vi "01b-add_two_numbers.vi"() -> ()   [LabVIEW 2018, in "LV-0mq-Julia_roundtrip-lib.lvlib"]
uses:
  LV-0mq-Julia_roundtrip-lib.lvlib
  Server or client state.ctl
  detailed error info.ctl
  StackFrame.ctl
  Commands.ctl
  d2cb43a9-9305-42fb-ad58-bce983510195.vi
  d2cb43a9-9305-42fb-ad58-bce983510195.vi/e28c4e1c-617d-4a26-8291-f58a5accd33d.vi
  d2cb43a9-9305-42fb-ad58-bce983510195.vi/697b26af-9cff-4296-98ec-fa9d12ca8fdc.vi
  d2cb43a9-9305-42fb-ad58-bce983510195.vi/17159f77-75f5-4b7b-8d47-844af2eb1bcd.vi
  jl-scripts path.vi
  check ID validity.vi
  bindata_descr to JSON.vi
  check cluster field names.vi
  concat JSON.vi
panel:
  in  "y":dbl=2.0
  in  "x":dbl=2.0
  in  "next":bool
  out "x+y":dbl=nan
  out "detailed error info":T1
  out "current error":errorcluster
  out "final error":errorcluster
  out "short err code":u8
  in  "stop":bool
  out "ZMQ timeout":bool
  out "Julia script file path":path
  out "temporary script path":path
  out "Jl Server state":T3
  # "This VI is slightly different from the previous example (see the wiring diagramm), but uses the same julia script."
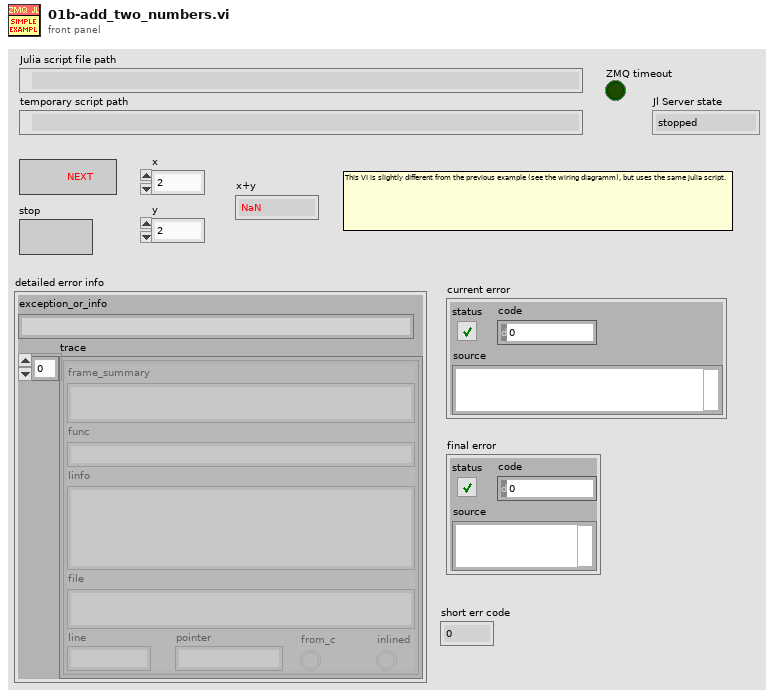
[diagram p1: front panel]
types:
  T1 = typedef "LV-0mq-Julia_roundtrip-lib.lvlib/detailed error info.ctl" = cluster{"exception_or_info":string, "trace":T2[]}
  T2 = typedef "LV-0mq-Julia_roundtrip-lib.lvlib/StackFrame.ctl" = cluster{"frame_summary":string, "func":string, "linfo":string, "file":string, "line":i32, "pointer":u64, "from_c":bool, "inlined":bool}
  T3 = typedef "LV-0mq-Julia_roundtrip-lib.lvlib/Server or client state.ctl" = enum16{"stopped", "running", "unknown"}
  T4 = typedef "LV-0mq-Julia_roundtrip-lib.lvlib/Commands.ctl" = enum16{"Start Jl-server & Init LV-client", "Send request & Get response ", "Stop Jl-server & Cleanup LV-client", "Cleanup LV-client", "Start Jl-server", "Stop Jl-server", "Init LV-Client", "Cleanup LV-Client", "(not allowed)", "Set LV Client state", "Set Jl Server state", "set ZMQ timeout", "read ZMQ timeout", "read-out state"}
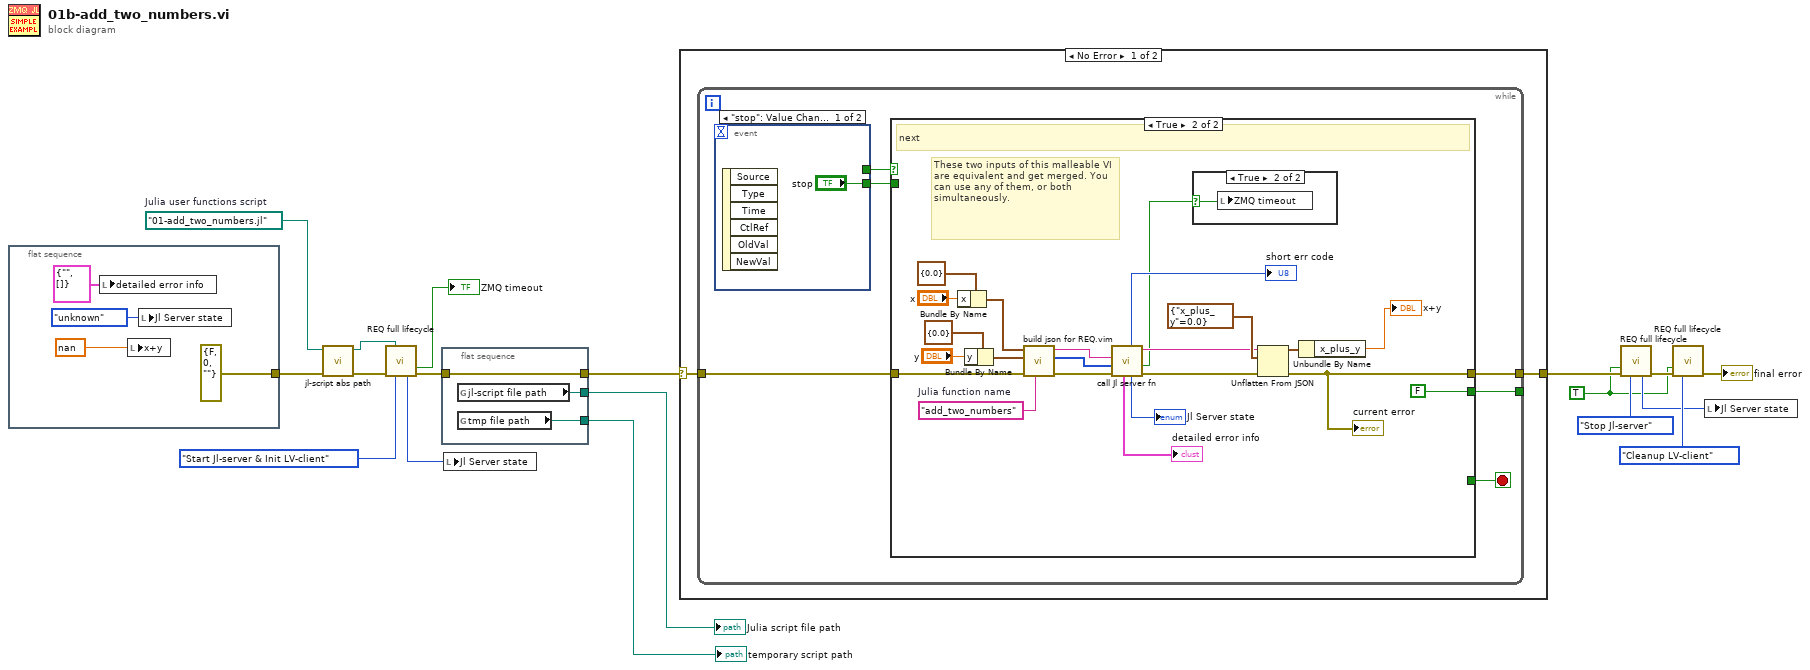
[diagram p0: block diagram]
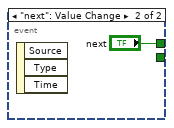
[diagram p2: hidden frame]
diagram:
  w4 = path "01-add_two_numbers.jl"  # Julia user functions script
  w1 = TRUE ("Force command")
  n1 = flat-sequence {
    tunnel: [errorcluster {"status"=FALSE, "code"=0, "source"=""} ("error in (no error)")] -> w2
    frame #0 {
      n2 = local write "detailed error info"(T1 {"exception_or_info"="", "trace"=[]} ("detailed error info")) -> ()
      n3 = local write "x+y"(nan ("Server response")) -> ()
      n4 = local write "Jl Server state"(Server_or_client_state."unknown" ("Jl Server state out")) -> ()
    }
  }
  n5 = call "jl-script abs path.vi"("error in (no error)"=w2, "Julia user functions script"=w4) -> ("error out"=w5:errorcluster, "script abs path"=w6:path)  [unwired: 8 in]
  n6 = call "REQ full lifecycle.vi"("Julia user functions script"=w6, "error in"=w5, "command"=Commands."Start Jl-server & Init LV-client") -> ("timeout?"=→"ZMQ timeout":bool, "Jl Server state out"=w8:T3, "error out"=w7:errorcluster)  [unwired: 6 in, 4 out]
  n7 = flat-sequence {
    tunnel: [w25] -> w13
    tunnel: w7 -> [w25]
    tunnel: [w24] -> w11
    tunnel: [w23] -> w12
    frame #0 {
      n8 = global read "jl-scripts path.vi" "jl-script file path"() -> (w24:path)
      n9 = global read "jl-scripts path.vi" "tmp file path"() -> (w23:path)
    }
  }
  n10 = local write "Jl Server state"(w8) -> ()
  n11 = case shown="No Error" w13 {
    selector: w13 -> [w26 w61]
    tunnel: [w27 w61] -> w18
    frame No Error {
      n12 = while {
        tunnel: w26 -> [w32]
        tunnel: [w33] -> w27
        tunnel: [w29] -> _
        stop <- w30 stop-if-true
        n13 = event shown="[0] \"stop\": Value Change" {
          selector: _ -> [_ _]
          dyn-events: _ -> [_ _]
          timeout: _ -> [_ _]
          tunnel: [_ "next"] -> w31
          tunnel: ["stop" _] -> w28
          event "stop": Value Change {
            n14 = event-data() -> ()  [unwired: 1 in, 6 out]
          }
          event "next": Value Change {
            n15 = event-data() -> ()  [unwired: 1 in, 3 out]
          }
        }
        n16 = case shown="True" w31 {
          tunnel: [w37 w55] -> w33
          tunnel: w32 -> [w37 w57]
          tunnel: [w36 w56] -> w30
          tunnel: [w36 w56] -> w29
          tunnel: w28 -> [w36 _]
          frame False {
            # "stop"
          }
          frame True {
            w44 = "add_two_numbers"  # Julia function name
            w56 = FALSE ("stop this VI only")
            # "These two inputs of this malleable VI are equivalent and get merged. You can use any of them, or both simultaneously."
            # "next"
            n17 = Bundle By Name(cluster=cluster{"x":dbl} {"x"=0.0}, "x"="x") -> (w41:cluster{"x":dbl})
            n18 = Bundle By Name(cluster=cluster{"y":dbl} {"y"=0.0}, "y"="y") -> (w38:cluster{"y":dbl})
            n19 = call "build json for REQ.vim"("fun2call"=w44, "error in (no error)"=w57, "Arguments 2"=w38, "Arguments 1"=w41) -> ("error out"=w51:errorcluster, "bindata out"=w52:u8[], "JSON string out"=w53:string)  [unwired: 5 in]
            n20 = call "call Jl server fn.vi"("error in (no error)"=w51, "binary data in"=w52, "JSON string in"=w53) -> ("error out"=w46:errorcluster, "timeout?"=w45:bool, "JSON received"=w48:string, "Jl Server state out"=→"Jl Server state":T3, "return code"=→"short err code":u8, "detailed error info"=→"detailed error info":T1)  [unwired: 2 in, 1 out]
            n21 = case shown="True" w45 {
              selector: w45 -> [_ w60]
              frame False {
              }
              frame True {
                n22 = local write "ZMQ timeout"(w60) -> ()
              }
            }
            n23 = Unflatten From JSON(JSON string=w48, type and defaults=cluster{"x_plus_y":dbl} {"x_plus_y"=0.0} ("parsed response"), error in (no error)=w46) -> (value=w58:cluster{"x_plus_y":dbl}, error out=w55:errorcluster)  [unwired: 4 in]
            "current error" <- w55
            n24 = Unbundle By Name(w58) -> ("x_plus_y"=→"x+y":dbl)
          }
        }
      }
    }
    frame Error {
    }
  }
  n25 = call "REQ full lifecycle.vi"("Force command"=w1, "error in"=w18, "command"=Commands."Stop Jl-server") -> ("Jl Server state out"=w10:T3, "error out"=w16:errorcluster)  [unwired: 6 in, 5 out]
  n26 = call "REQ full lifecycle.vi"("Force command"=w1, "error in"=w16, "command"=Commands."Cleanup LV-client") -> ("error out"=→"final error":errorcluster)  [unwired: 6 in, 6 out]
  n27 = local write "Jl Server state"(w10) -> ()
  "temporary script path" <- w12
  "Julia script file path" <- w11
